vi "Read ADU.vi"(8 "error in (no error)":errorcluster, 11 "MB_Serial_Master in":refnum<class "MB_Master_Serial.lvclass">) -> (0 "error out":errorcluster, 2 "MB_ADU":refnum<class "MB_ADU.lvclass">, 3 "MB_Serial_Master out":refnum<class "MB_Master_Serial.lvclass">)   [LabVIEW 2012, in "MB Master.lvlib" / "MB_Master_Serial.lvclass"]
uses:
  MB_Master_Serial.lvclass
  MB_ADU/MB_ADU.lvclass
  MB_Master_Serial.lvclass/MB_Master_Serial.ctl
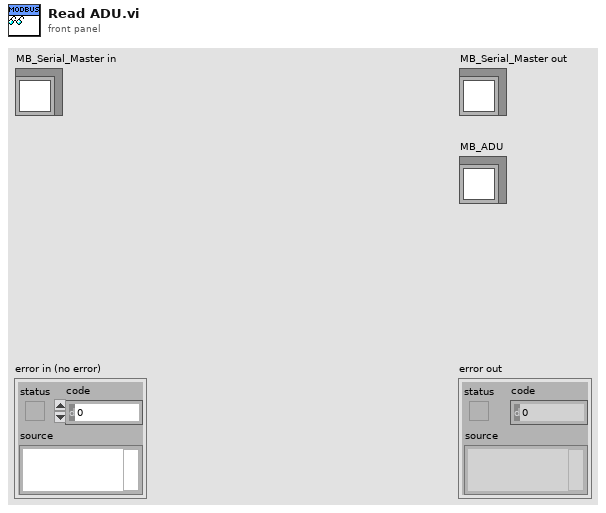
[diagram p1: front panel]
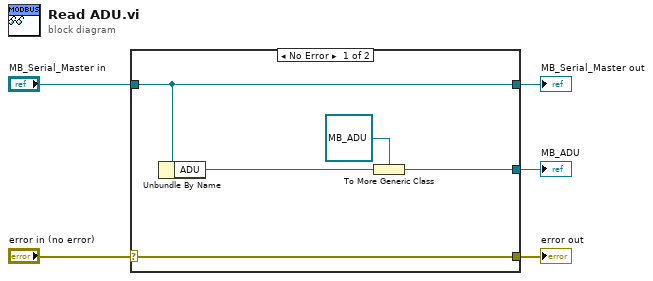
[diagram p0: block diagram]
diagram:
  n1 = case shown="No Error" "error in (no error)" {
    selector: "error in (no error)" -> [w10 w11]
    tunnel: [w10 w11] -> w4
    tunnel: [w9 w12] -> w2
    tunnel: "MB_Serial_Master in" -> [w9 w12]
    tunnel: [w6 _] -> w1
    frame No Error {
      n2 = Unbundle By Name(w9) -> ("ADU"=w7:refnum<class "MB_ADU_Serial.lvclass">)
      n3 = To More Generic Class(target class=refnum<class "MB_ADU.lvclass"> refnum ("MB_ADU"), reference=w7) -> (generic class reference=w6:refnum<class "MB_ADU.lvclass">)
    }
    frame Error {
    }
  }
  "error out" <- w4
  "MB_Serial_Master out" <- w2
  "MB_ADU" <- w1
